vi "Initialize, has to run once.vi"() -> ()   [LabVIEW 2014]
panel:
  in  "VISA Refnum in":refnum<visa-resource-name>
  in  "stop":bool
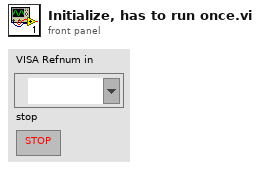
[diagram p1: front panel]
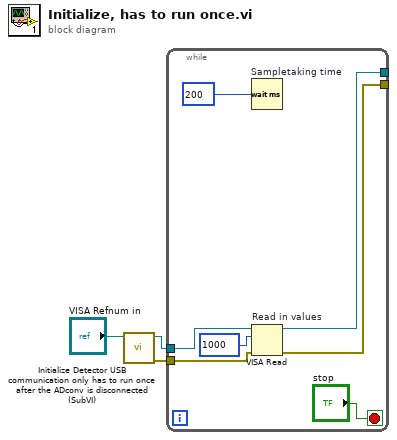
[diagram p0: block diagram]
diagram:
  n1 = call "Initialize Detector USB communication only has to run once after the ADconv is disconnected (SubVI).vi"("VISA Refnum in"="VISA Refnum in") -> ("error out"=w1:errorcluster, "VISA Refnum out"=w2:refnum<visa-resource-name>)  [unwired: 7 in, 2 out]
  n2 = while {
    tunnel: w2 -> [w9]
    tunnel: [w8] -> _
    tunnel: [w7] -> _
    tunnel: w1 -> [w6]
    stop <- "stop" stop-if-true
    n3 = Wait (ms) "Sampletaking time"(milliseconds to wait=u32 200 ("millisecond timer value")) -> ()  [unwired: 1 out]
    n4 = VISA Read "Read in values"(VISA resource name=w9, byte count=u32 1000, error in (no error)=w6) -> (VISA resource name out=w7:refnum<visa-resource-name>, error out=w8:errorcluster)  [unwired: 2 out]
  }
